vi "PI Convert 1.5 to 1.6.vi"(0 "Prompted Inputs 1.5 Test Parameters":T2) -> (2 "Prompted Inputs 1.6 Test Parameters":T1)   [LabVIEW 2011]
uses:
  TypeDefs/PI Test Parameters v1.5.ctl
  TypeDefs/PI Test Parameters v1.6.ctl
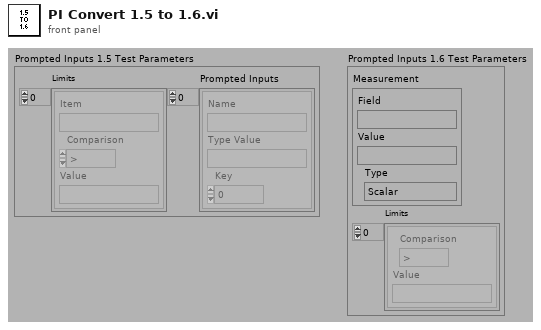
[diagram p1: front panel]
types:
  T1 = typedef "PI Test Parameters v1.6.ctl" = cluster{"Measurement":cluster{"Field":string, "Value":string, "Type":enum16{"Scalar", "Enumeration"}}, "Limits":cluster{"Comparison":enum16{">", ">=", "<", "<=", "<>", "="}, "Value":string}[]}
  T2 = typedef "PI Test Parameters v1.5.ctl" = cluster{"Limits":cluster{"Item":string, "Comparison":enum16{">", ">=", "<", "<=", "<>", "="}, "Value":string}[], "Prompted Inputs":cluster{"Name":string, "Type Value":string, "Key":i32}[]}
  T3 = cluster{"Item":string, "Comparison":enum16{">", ">=", "<", "<=", "<>", "="}, "Value":string}[]
  T4 = cluster{"Name":string, "Type Value":string, "Key":i32}[]
  T5 = cluster{"Name":string, "Type Value":string, "Key":i32}
  T6 = cluster{"Comparison":enum16{">", ">=", "<", "<=", "<>", "="}, "Value":string}[]
  T7 = cluster{"Comparison":enum16{">", ">=", "<", "<=", "<>", "="}, "Value":string}
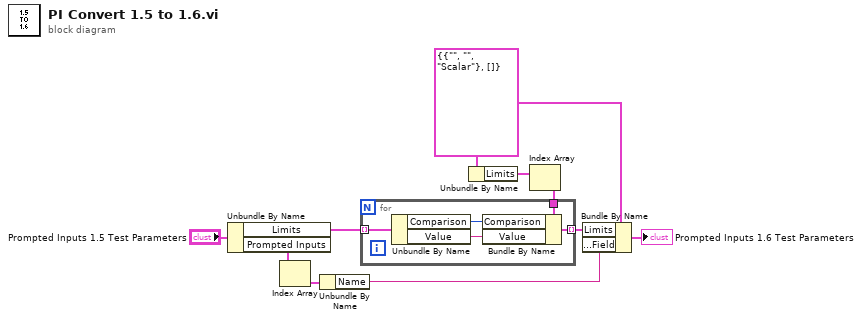
[diagram p0: block diagram]
diagram:
  w1 = T1 {"Measurement"={"Field"="", "Value"="", "Type"=enum."Scalar"}, "Limits"=[]} ("Prompted Inputs Test Parameters")
  n1 = Unbundle By Name("Prompted Inputs 1.5 Test Parameters") -> ("Limits"=w5:T3, "Prompted Inputs"=w8:T4)
  n2 = Index Array(array=w8) -> (element=w7:T5)  [unwired: 1 in]
  n3 = Unbundle By Name(w7) -> ("Name"=w6:string)
  n4 = Unbundle By Name(w1) -> ("Limits"=w4:T6)
  n5 = Index Array(array=w4) -> (element=w3:T7)  [unwired: 1 in]
  n6 = for {
    tunnel: w5 -> [w15] mode=indexing
    tunnel: w3 -> [w14]
    tunnel: [w11] -> w2 mode=indexing
    n7 = Unbundle By Name(w15) -> ("Comparison"=w13:enum16{">", ">=", "<", "<=", "<>", "="}, "Value"=w12:string)
    n8 = Bundle By Name(cluster=w14, "Comparison"=w13, "Value"=w12) -> (w11:T7)
  }
  n9 = Bundle By Name(cluster=w1, "Limits"=w2, "Measurement.Field"=w6) -> (→"Prompted Inputs 1.6 Test Parameters":T1)
